vi "CRON.CreateBroadcasts.vi"(8 "error in (no error)":errorcluster) -> (0 "error out":errorcluster, 3 "Broadcasts":T1)   [LabVIEW 2024, in "CRON.lvclass"]
uses:
  CRON.lvclass
  CRON.lvclass/CRON.ctl
  Stopped.ctl
  Broadcast Events--cluster.ctl
  RQMHCore/ModuleCore/RQMHModule.lvclass
  Fired.ctl
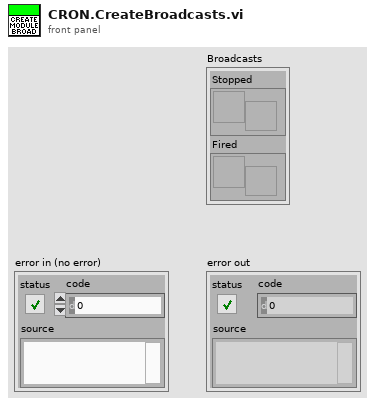
[diagram p1: front panel]
types:
  T1 = typedef "CRON.lvclass/Broadcast Events--cluster.ctl" = cluster{"Stopped":refnum<user-event>, "Fired":refnum<user-event>}
  T2 = typedef "CRON.lvclass/Fired.ctl" = cluster{"Module":refnum<class "RQMHModule.lvclass">}
  T3 = typedef "CRON.lvclass/Stopped.ctl" = bool
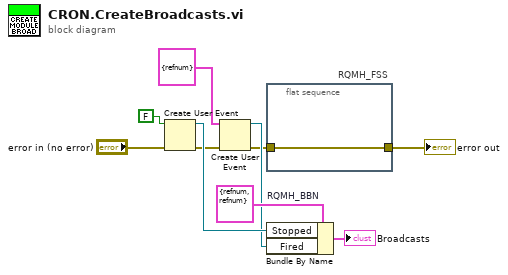
[diagram p0: block diagram]
diagram:
  n1 = Create User Event(user event datatype=T3 FALSE ("Stopped"), error in="error in (no error)") -> (user event=w9:refnum<user-event>, error out=w1:errorcluster)
  n2 = Create User Event(user event datatype=T2 {"Module"=refnum} ("Fired"), error in=w1) -> (user event=w3:refnum<user-event>, error out=w2:errorcluster)
  n3 = flat-sequence "RQMH_FSS" {
    tunnel: w2 -> [w11]
    tunnel: [w11] -> w5
    frame #0 {
    }
  }
  n4 = Bundle By Name "RQMH_BBN"(cluster=T1 {"Stopped"=refnum, "Fired"=refnum} ("Broadcasts"), "Stopped"=w9, "Fired"=w3) -> (→"Broadcasts":T1)
  "error out" <- w5
